vi "Error Converter (ErrCode or Status).vi"(8 "error in (no error)":errorcluster caption="entrée d'erreur (pas d'erreur)", 11 "error code":i32 caption="code d'erreur") -> (0 "error out":errorcluster caption="sortie d'erreur")   [LabVIEW 2020, in "Library Instrument & Equipement.lvlib" / "Library Printer.lvlib" / "TSCLIB.lvlib"]
uses:
  TSCLIB.lvlib
panel:
  in  "string":string="Cette erreur est renvoyée par la fonction de la bibliothèque partagée." caption="chaîne"
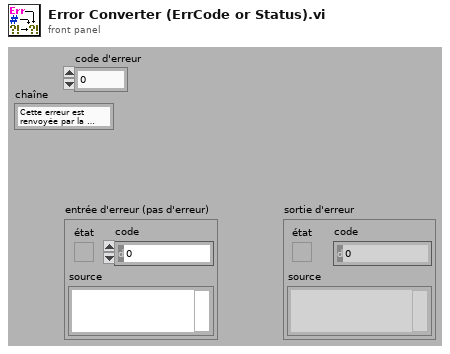
[diagram p1: front panel]
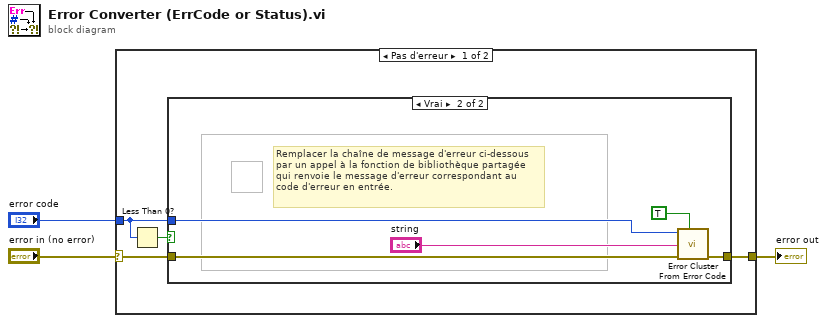
[diagram p0: block diagram]
diagram:
  n1 = case shown="Pas d'erreur" "error in (no error)" {
    selector: "error in (no error)" -> [w6 w14]
    tunnel: [w4 w14] -> w2
    tunnel: "error code" -> [w5 _]
    frame No Error {
      n2 = Less Than 0?(x=w5) -> (x < 0?=w7:bool)
      n3 = case shown="Vrai" w7 {
        tunnel: w6 -> [w8 w13]
        tunnel: w5 -> [_ w11]
        tunnel: [w8 w12] -> w4
        frame False {
        }
        frame True {
          # "Remplacer la chaîne de message d'erreur ci-dessous par un appel à la fonction de bibliothèque partagée qui renvoie le message d'erreur correspondant au code d'erreur en entrée."
          n4 = call <vilib>:"Error Cluster From Error Code.vi"("show call chain? (False)"=TRUE, "error in (no error)"=w13, "error message (\"\")"="string", "error code (0)"=w11) -> ("error out"=w12:errorcluster)  [unwired: 5 in]
        }
      }
    }
    frame Error {
    }
  }
  "error out" <- w2
